vi "A1 处理函数.vi"(8 "error in (no error)":errorcluster caption="错误输入（无错误）", 9 "Session Out":T2, 10 "Image Name":string="I1", 11 "ParamsUI":T1 caption="参数界面" {"Exposure Values" scale=0.0..200000.0}) -> (0 "error out":errorcluster caption="错误输出", 3 "Image out":T3(plugin-control))   [LabVIEW 2017]
uses:
  <vilib>/userdefined/High Color/IMAQdx.ctl
  <resource>/objmgr/imaqdx.rc
  <vilib>/vision/driver/NI_Vision_Acquisition_Software.lvlib
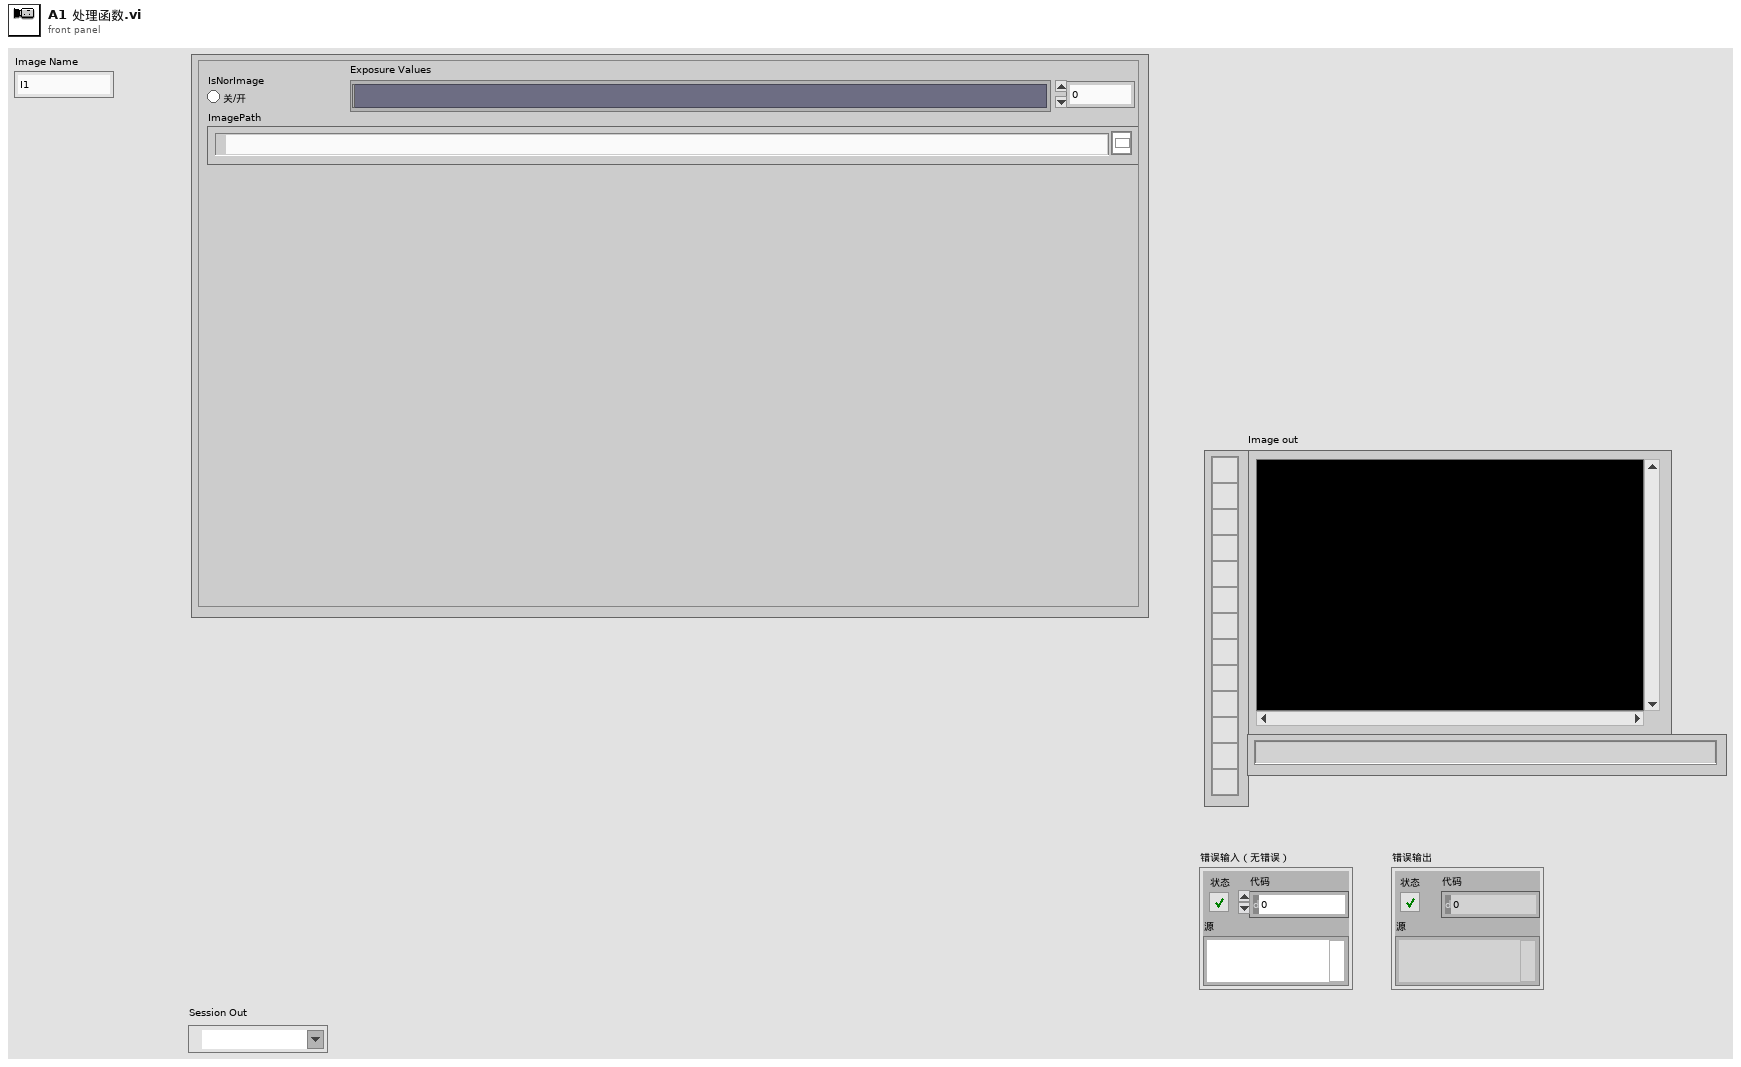
[diagram p1: front panel]
types:
  T1 = cluster{"IsNorImage":bool, "Exposure Values":u32, "ImagePath":path}
  T2 = typedef "IMAQdx.ctl" = refnum<k21>
  T3 = typedef "IMAQ Image.ctl" = refnum<image>
  T4 = typedef "Image Type" = u32
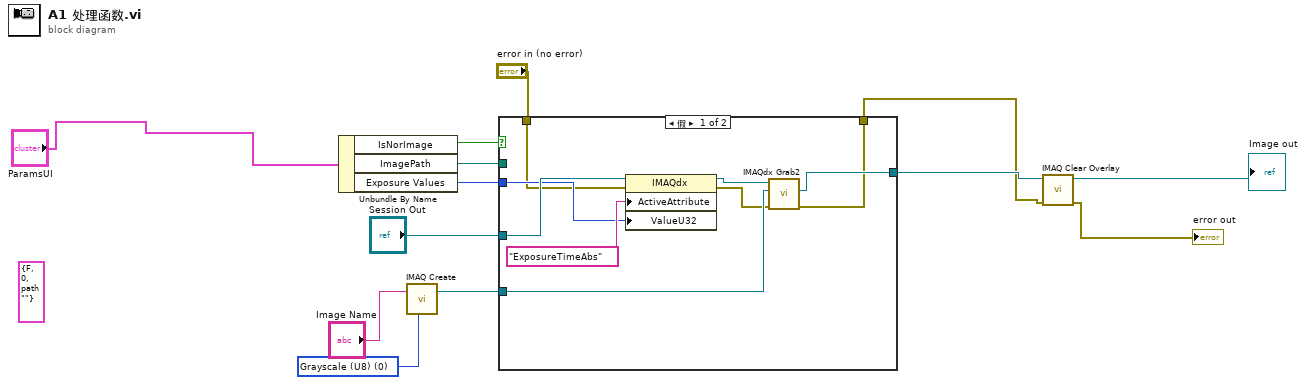
[diagram p0: block diagram]
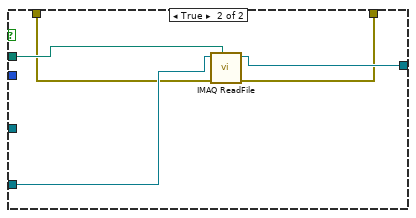
[diagram p2: hidden frame]
diagram:
  w5 = T4 0 items=["Grayscale (U8)", "Grayscale (I16)", "Grayscale (SGL)", "Complex (CSG)", "RGB (U32)", "HSL (U32)", "RGB (U64)", "Grayscale (U16)"] ("Image Type")
  (unwired) T1 {"IsNorImage"=FALSE, "Exposure Values"=0, "ImagePath"=path ""} ("ParamsUI")
  n1 = Unbundle By Name("ParamsUI") -> ("IsNorImage"=w13:bool, "ImagePath"=w12:path, "Exposure Values"=w11:u32)
  n2 = call "IMAQ Create"("Image Name"="Image Name", "Image Type"=w5) -> ("New Image"=w8:T3)  [unwired: 3 in, 1 out]
  n3 = case shown="假" w13 {
    tunnel: w12 -> [_ w27]
    tunnel: [w16 w26] -> w4
    tunnel: w11 -> [w20 _]
    tunnel: "Session Out" -> [w22 _]
    tunnel: w8 -> [w18 w25]
    tunnel: "error in (no error)" -> [w15 w24]
    tunnel: [w14 w23] -> w3
    frame False {
      n4 = property class="IMAQdx"(reference=w22, error in=w15, "ActiveAttribute"="ExposureTimeAbs", "ValueU32"=w20) -> (reference out=w19:T2, error out=w17:errorcluster)
      n5 = call <vilib>:"IMAQdx Grab2.vi"("error in"=w17, "Image In"=w18, "Session In"=w19) -> ("error out"=w14:errorcluster, "Image Out"=w16:T3)  [unwired: 5 in, 2 out]
    }
    frame True {
      n6 = call "IMAQ ReadFile"("File Path"=w27, "error in (no error)"=w24, "Image"=w25) -> ("error out"=w23:errorcluster, "Image Out"=w26:T3)  [unwired: 4 in, 3 out]
    }
  }
  n7 = call "IMAQ Clear Overlay"("error in (no error)"=w3, "Image"=w4) -> ("error out"=→"error out":errorcluster, "Image Out"=→"Image out":T3)  [unwired: 8 in]
